vi "CRYAPI TAB LIB.vi"(8 "tPage":T1, 9 "tFrame":T3, 10 "nData":i32, 11 "sAction":string) -> (0 "nData_Out":i32, 2 "tFrame_Out":T3, 3 "tPage_Out":T1)   [LabVIEW 2013]
uses:
  <vilib>/Utility/miscctls.llb/LVRectTypeDef.ctl
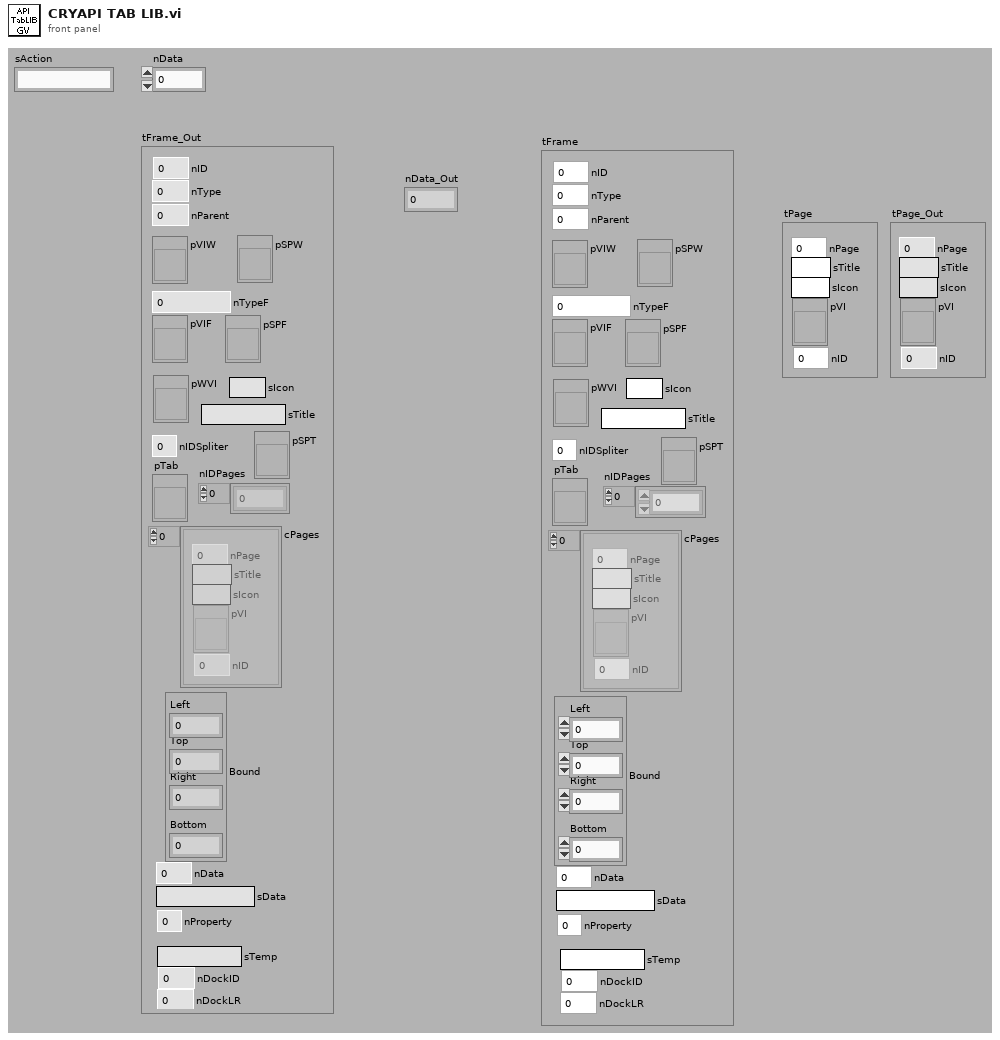
[diagram p1: front panel]
types:
  T1 = cluster{"nPage":i32, "sTitle":string, "sIcon":string, "pVI":refnum<vi>, "nID":i32}
  T2 = typedef "LVRectTypeDef.ctl" = cluster{"Left":i16, "Top":i16, "Right":i16, "Bottom":i16}
  T3 = cluster{"nType":i32, "nParent":i32, "pVIW":refnum<vi>, "pSPW":refnum<vi>, "nTypeF":i32, "pVIF":refnum<vi>, "pSPF":refnum<vi>, "nIDSpliter":i32, "nProperty":i32, "Bound":T2, "nID":i32, "nData":i32, "sData":string, "pWVI":refnum<vi>, "sTitle":string, "cPages":cluster{"nPage":i32, "sTitle":string, "sIcon":string, "pVI":refnum<vi>, "nID":i32}[], "pTab":refnum<vi>, "nIDPages":i32[], "pSPT":refnum<vi>, "sTemp":string, "nDockID":i32, "nDockLR":i32, "sIcon":string}
  T4 = cluster{"nPage":i32, "sTitle":string, "sIcon":string, "pVI":refnum<vi>, "nID":i32}[]
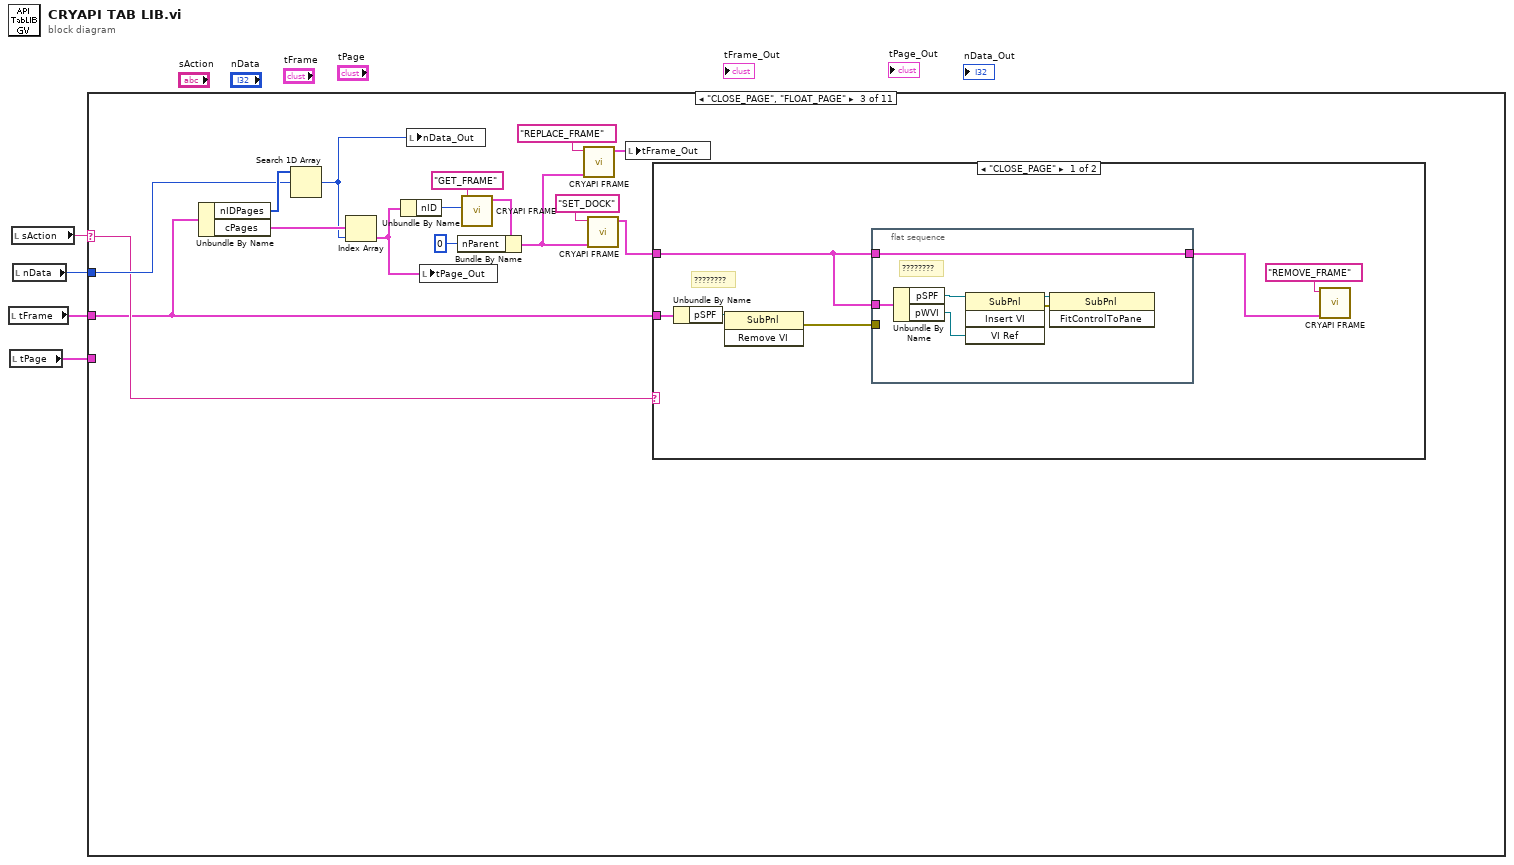
[diagram p0: block diagram]
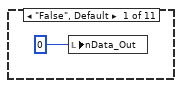
[diagram p2: hidden frame]
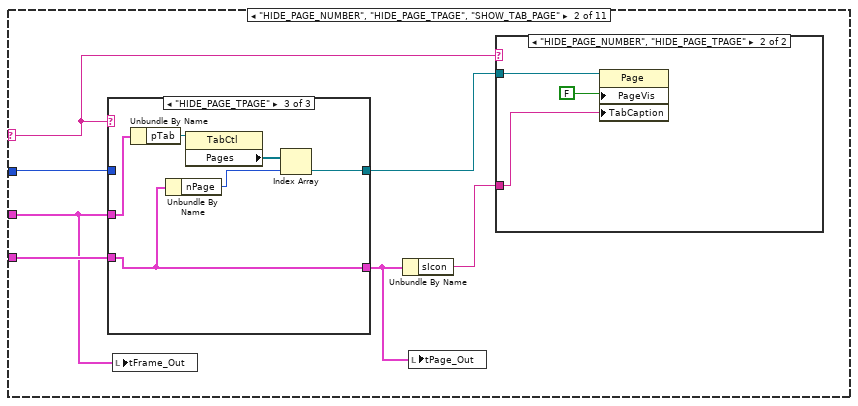
[diagram p3: hidden frame]
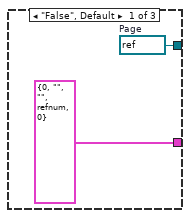
[diagram p4: hidden frame]
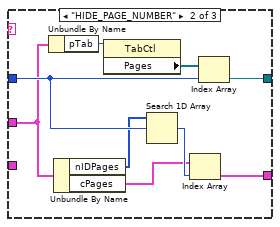
[diagram p5: hidden frame]
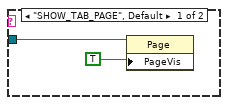
[diagram p6: hidden frame]
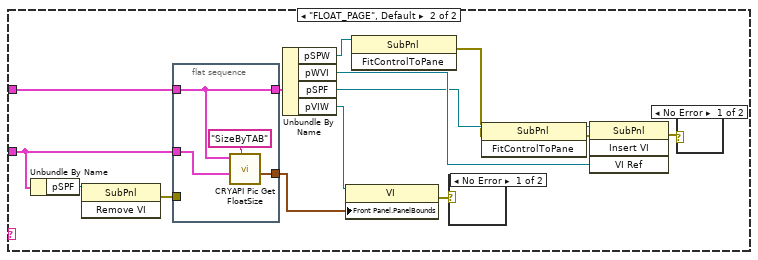
[diagram p7: hidden frame]
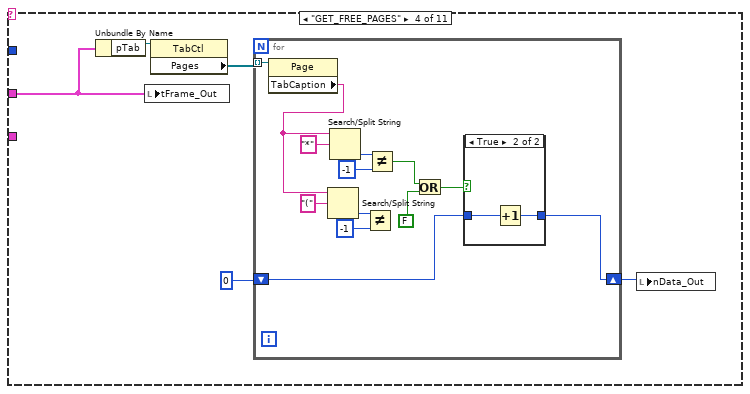
[diagram p10: hidden frame]
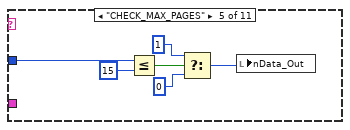
[diagram p12: hidden frame]
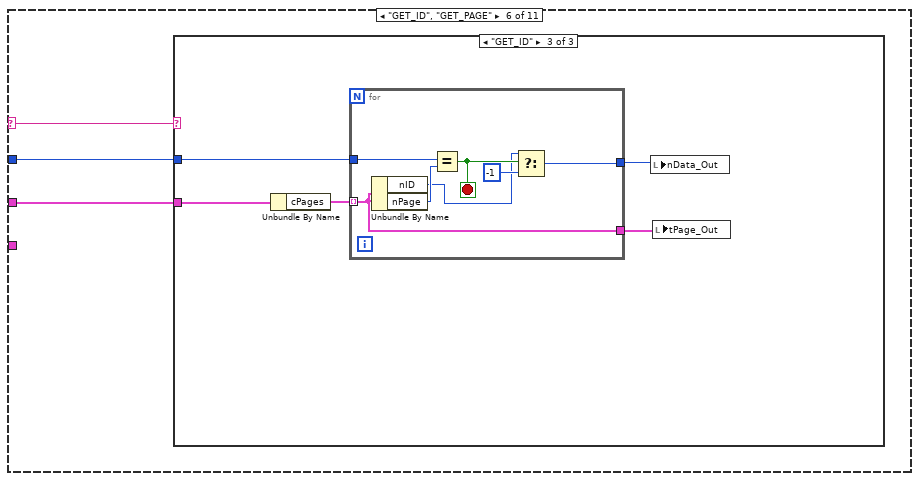
[diagram p13: hidden frame]
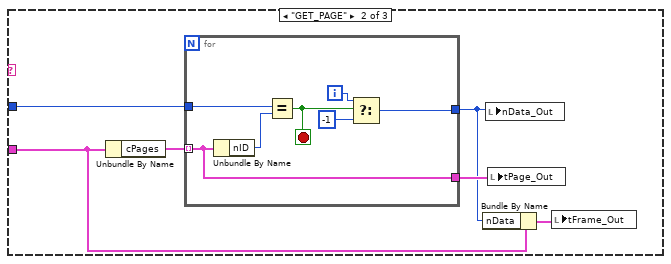
[diagram p15: hidden frame]
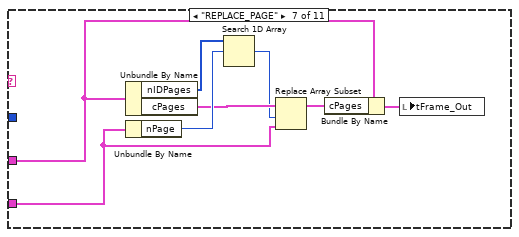
[diagram p16: hidden frame]
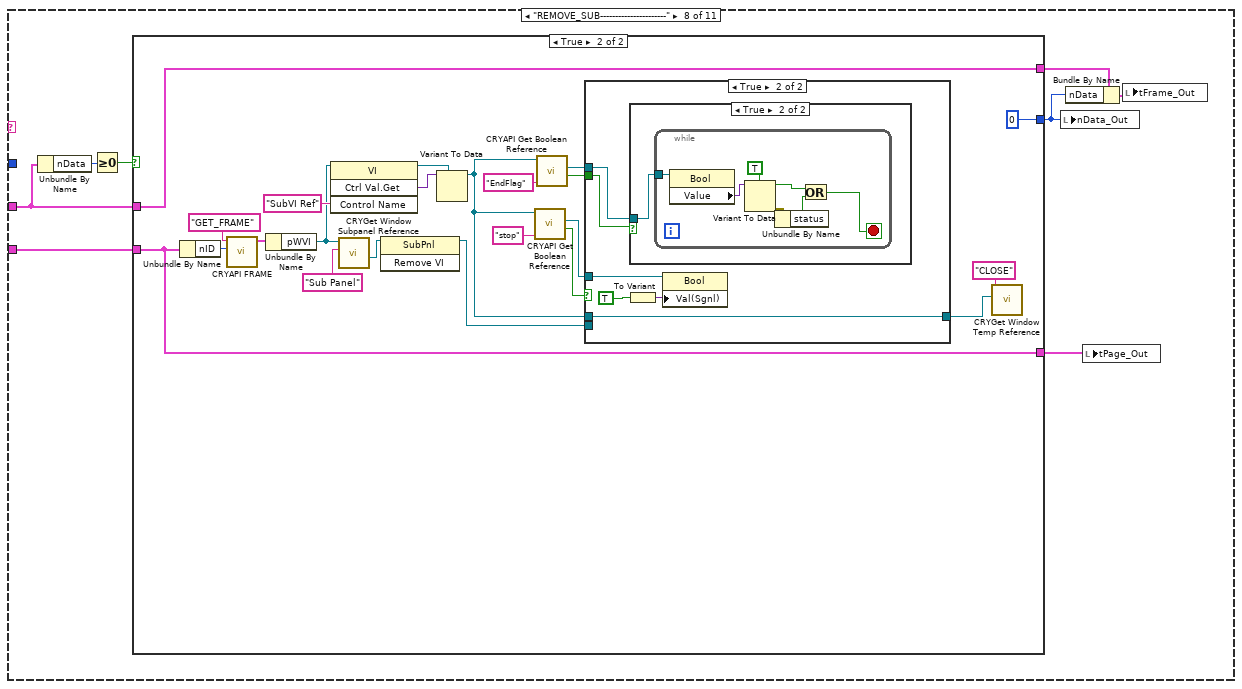
[diagram p17: hidden frame]
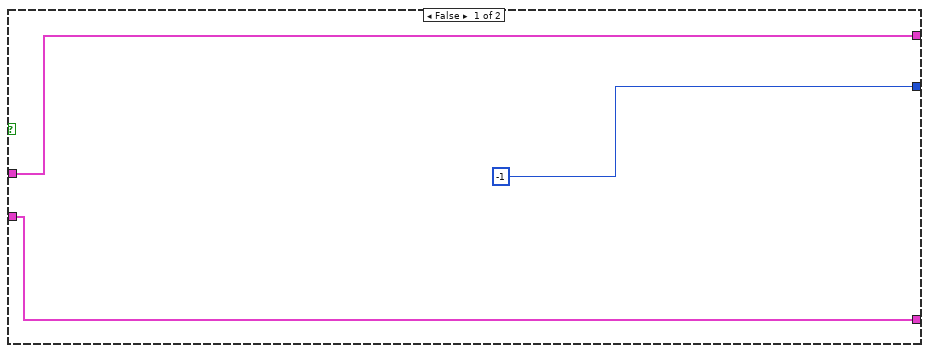
[diagram p18: hidden frame]
diagram:
  n1 = local read "tFrame"() -> (w3:T3)
  n2 = local read "tPage"() -> (w2:T1)
  n3 = local read "sAction"() -> (w4:string)
  n4 = local read "nData"() -> (w1:i32)
  n5 = case shown="\"CLOSE_PAGE\", \"FLOAT_PAGE\"" w4 {
    selector: w4 -> [_ w8 w40 _ _ w109 _ _ _ _ _]
    tunnel: w3 -> [_ w6 w35 w82 _ w110 w142 w146 w194 w258 w288]
    tunnel: w2 -> [_ w7 _ _ _ _ w139 w151 w197 _ _]
    tunnel: w1 -> [_ w11 w47 _ w108 w111 _ _ _ w257 _]
    frame "False", Default {
      n6 = local write "nData_Out"(0 ("nData_Out")) -> ()
    }
    frame "HIDE_PAGE_NUMBER", "HIDE_PAGE_TPAGE", "SHOW_TAB_PAGE" {
      n7 = case shown="\"HIDE_PAGE_TPAGE\"" w8 {
        tunnel: [w14 w21 w27] -> w12
        tunnel: w11 -> [_ w20 _]
        tunnel: [T1 {"nPage"=0, "sTitle"="", "sIcon"="", "pVI"=refnum, "nID"=0} ("tPage") w19 w26] -> w9
        tunnel: w7 -> [_ _ w26]
        tunnel: w6 -> [_ w15 w24]
        frame "False", Default {
          w14 = refnum<vi> refnum  # Page
        }
        frame "HIDE_PAGE_NUMBER" {
          n8 = Unbundle By Name(w15) -> ("pTab"=w23:refnum<vi>)
          n9 = Unbundle By Name(w15) -> ("nIDPages"=w18:i32[], "cPages"=w16:T4)
          n10 = property class="TabCtl"(reference=w23) -> ("Pages"=w22:refnum<vi>[])  [unwired: 1 in, 2 out]
          n11 = Search 1D Array(1D array=w18, element=w20) -> (index of element=w17:i32)  [unwired: 1 out]
          n12 = Index Array(array=w16, index=w17) -> (element=w19:T1)
          n13 = Index Array(array=w22, index=w20) -> (element=w21:refnum<vi>)
        }
        frame "HIDE_PAGE_TPAGE" {
          n14 = Unbundle By Name(w24) -> ("pTab"=w29:refnum<vi>)
          n15 = Unbundle By Name(w26) -> ("nPage"=w25:i32)
          n16 = property class="TabCtl"(reference=w29) -> ("Pages"=w28:refnum<vi>[])  [unwired: 1 in, 2 out]
          n17 = Index Array(array=w28, index=w25) -> (element=w27:refnum<vi>)
        }
      }
      n18 = local write "tFrame_Out"(w6) -> ()
      n19 = Unbundle By Name(w9) -> ("sIcon"=w10:string)
      n20 = local write "tPage_Out"(w9) -> ()
      n21 = case shown="\"HIDE_PAGE_NUMBER\", \"HIDE_PAGE_TPAGE\"" w8 {
        tunnel: w12 -> [w30 w33]
        tunnel: w10 -> [_ w32]
        frame "SHOW_TAB_PAGE", Default {
          n22 = property class="Page"(reference=w30, "PageVis"=TRUE ("Page Visible")) -> ()  [unwired: 1 in, 2 out]
        }
        frame "HIDE_PAGE_NUMBER", "HIDE_PAGE_TPAGE" {
          n23 = property class="Page"(reference=w33, "PageVis"=FALSE ("Page Visible"), "TabCaption"=w32) -> ()  [unwired: 1 in, 2 out]
        }
      }
    }
    frame "CLOSE_PAGE", "FLOAT_PAGE" {
      n24 = Unbundle By Name(w35) -> ("nIDPages"=w49:i32[], "cPages"=w48:T4)
      n25 = Search 1D Array(1D array=w49, element=w47) -> (index of element=w37:i32)  [unwired: 1 out]
      n26 = Index Array(array=w48, index=w37) -> (element=w45:T1)
      n27 = Unbundle By Name(w45) -> ("nID"=w46:i32)
      n28 = local write "nData_Out"(w37) -> ()
      n29 = local write "tPage_Out"(w45) -> ()
      n30 = call "CRYAPI FRAME.vi"("nData"=w46, "sAction"="GET_FRAME") -> ("tFrame_Out"=w44:T3)  [unwired: 4 in, 5 out]
      n31 = Bundle By Name(cluster=w44, "nParent"=0) -> (w38:T3)
      n32 = call "CRYAPI FRAME.vi"("tFrame"=w38, "sAction"="REPLACE_FRAME") -> ("tFrame_Out"=w41:T3)  [unwired: 4 in, 5 out]
      n33 = call "CRYAPI FRAME.vi"("tFrame"=w38, "sAction"="SET_DOCK") -> ("tFrame_Out"=w36:T3)  [unwired: 4 in, 5 out]
      n34 = local write "tFrame_Out"(w41) -> ()
      n35 = case shown="\"CLOSE_PAGE\"" w40 {
        tunnel: w36 -> [w55 w75]
        tunnel: w35 -> [w52 w76]
        frame "CLOSE_PAGE" {
          # "????????"
          n36 = Unbundle By Name(w52) -> ("pSPF"=w53:refnum<vi>)
          n37 = invoke class="SubPnl" method="Remove VI"(reference=w53) -> (error out=w51:errorcluster)  [unwired: 2 in, 2 out]
          n38 = flat-sequence {
            tunnel: w55 -> [w62]
            tunnel: w55 -> [w57]
            tunnel: [w57] -> w54
            tunnel: w51 -> [_]
            frame #0 {
              # "????????"
              n39 = Unbundle By Name(w62) -> ("pSPF"=w59:refnum<vi>, "pWVI"=w58:refnum<vi>)
              n40 = invoke class="SubPnl" method="Insert VI"(reference=w59, "VI Ref"=w58) -> (reference out=w61:refnum<vi>, error out=w60:errorcluster)  [unwired: 2 in, 2 out]
              n41 = invoke class="SubPnl" method="FitControlToPane"(reference=w61, error in=w60) -> ()  [unwired: 1 in, 3 out]
            }
          }
          n42 = call "CRYAPI FRAME.vi"("tFrame"=w54, "sAction"="REMOVE_FRAME") -> ()  [unwired: 4 in, 6 out]
        }
        frame "FLOAT_PAGE", Default {
          n43 = Unbundle By Name(w76) -> ("pSPF"=w77:refnum<vi>)
          n44 = invoke class="SubPnl" method="Remove VI"(reference=w77) -> (error out=w73:errorcluster)  [unwired: 2 in, 2 out]
          n45 = flat-sequence {
            tunnel: w76 -> [w81]
            tunnel: w75 -> [w78]
            tunnel: [w80] -> w74
            tunnel: w73 -> [_]
            tunnel: [w78] -> w72
            frame #0 {
              n46 = call "CRYAPI Pic Get FloatSize.vi"("sAction"="SizeByTAB", "tFrameTAB"=w81, "tFrame"=w78) -> ("FPPanelBound_Out"=w80:T2)  [unwired: 7 in, 1 out]
            }
          }
          n47 = Unbundle By Name(w72) -> ("pSPW"=w65:refnum<vi>, "pWVI"=w70:refnum<vi>, "pSPF"=w68:refnum<vi>, "pVIW"=w71:refnum<vi>)
          n48 = property class="VI"(reference=w71, "Front Panel.PanelBounds"=w74) -> (error out=w63:errorcluster)  [unwired: 1 in, 1 out]
          n49 = invoke class="SubPnl" method="FitControlToPane"(reference=w65) -> (error out=w64:errorcluster)  [unwired: 2 in, 2 out]
          n50 = case shown="No Error" w63 {
            frame No Error {
            }
            frame Error {
            }
          }
          n51 = invoke class="SubPnl" method="FitControlToPane"(reference=w68, error in=w64) -> (reference out=w67:refnum<vi>, error out=w66:errorcluster)  [unwired: 1 in, 1 out]
          n52 = invoke class="SubPnl" method="Insert VI"(reference=w67, error in=w66, "VI Ref"=w70) -> (error out=w69:errorcluster)  [unwired: 1 in, 3 out]
          n53 = case shown="No Error" w69 {
            frame No Error {
            }
            frame Error {
            }
          }
        }
      }
    }
    frame "GET_FREE_PAGES" {
      n54 = Unbundle By Name(w82) -> ("pTab"=w86:refnum<vi>)
      n55 = local write "tFrame_Out"(w82) -> ()
      n56 = property class="TabCtl"(reference=w86) -> ("Pages"=w85:refnum<vi>[])  [unwired: 1 in, 2 out]
      n57 = for {
        tunnel: w85 -> [w99] mode=indexing
        shift-right: [w88] -> w83
        shift-left: 0 -> [w89]
        n58 = property class="Page"(reference=w99) -> ("TabCaption"=w92:string)  [unwired: 1 in, 2 out]
        n59 = Search/Split String(string=w92, search string/char (-)="(") -> (offset of match=w95:i32)  [unwired: 3 out]
        n60 = Search/Split String(string=w92, search string/char (-)="*") -> (offset of match=w97:i32)  [unwired: 3 out]
        n61 = Not Equal?(x=w95, y=-1) -> ()  [unwired: 1 out]
        n62 = Not Equal?(x=w97, y=-1) -> (x != y?=w91:bool)
        n63 = Or(x=w91, y=FALSE) -> (x .or. y?=w90:bool)
        n64 = case shown="True" w90 {
          tunnel: w89 -> [w100 w102]
          tunnel: [w100 w101] -> w88
          frame False {
          }
          frame True {
            n65 = Increment(x=w102) -> (x+1=w101:i32)
          }
        }
      }
      n66 = local write "nData_Out"(w83) -> ()
    }
    frame "CHECK_MAX_PAGES" {
      n67 = Less Or Equal?(x=w108, y=15) -> (x <= y?=w106:bool)
      n68 = Select(t=1, s=w106, f=0) -> (s? t:f=w103:i32)
      n69 = local write "nData_Out"(w103) -> ()
    }
    frame "GET_ID", "GET_PAGE" {
      n70 = case shown="\"GET_ID\"" w109 {
        tunnel: w111 -> [_ w116 w128]
        tunnel: w110 -> [_ w114 w126]
        frame "False", Default {
        }
        frame "GET_PAGE" {
          n71 = Unbundle By Name(w114) -> ("cPages"=w117:T4)
          n72 = for {
            tunnel: w117 -> [w122] mode=indexing
            tunnel: w116 -> [w124]
            tunnel: [w122] -> w115
            tunnel: [w118] -> w113
            i -> [w120]
            stop <- w121 stop-if-true
            n73 = Unbundle By Name(w122) -> ("nID"=w123:i32)
            n74 = Equal?(x=w124, y=w123) -> (x = y?=w121:bool)
            n75 = Select(t=w120, s=w121, f=-1) -> (s? t:f=w118:i32)
          }
          n76 = Bundle By Name(cluster=w114, "nData"=w113) -> (w112:T3)
          n77 = local write "nData_Out"(w113) -> ()
          n78 = local write "tPage_Out"(w115) -> ()
          n79 = local write "tFrame_Out"(w112) -> ()
        }
        frame "GET_ID" {
          n80 = Unbundle By Name(w126) -> ("cPages"=w129:T4)
          n81 = for {
            tunnel: w129 -> [w134] mode=indexing
            tunnel: w128 -> [w136]
            tunnel: [w134] -> w127
            tunnel: [w131] -> w125
            stop <- w133 stop-if-true
            n82 = Unbundle By Name(w134) -> ("nID"=w130:i32, "nPage"=w135:i32)
            n83 = Equal?(x=w136, y=w135) -> (x = y?=w133:bool)
            n84 = Select(t=w130, s=w133, f=-1) -> (s? t:f=w131:i32)
          }
          n85 = local write "nData_Out"(w125) -> ()
          n86 = local write "tPage_Out"(w127) -> ()
        }
      }
    }
    frame "REPLACE_PAGE" {
      n87 = Unbundle By Name(w142) -> ("nIDPages"=w144:i32[], "cPages"=w141:T4)
      n88 = Unbundle By Name(w139) -> ("nPage"=w143:i32)
      n89 = Search 1D Array(1D array=w144, element=w143) -> (index of element=w140:i32)  [unwired: 1 out]
      n90 = Replace Array Subset(array=w141, new element=w139, index=w140) -> (w138:T4)
      n91 = Bundle By Name(cluster=w142, "cPages"=w138) -> (w137:T3)
      n92 = local write "tFrame_Out"(w137) -> ()
    }
    frame "REMOVE_SUB----------------------" {
      n93 = Unbundle By Name(w146) -> ("nData"=w145:i32)
      n94 = Greater Or Equal To 0?(x=w145) -> (x >= 0?=w152:bool)
      n95 = case shown="True" w152 {
        tunnel: w146 -> [w154 w176]
        tunnel: w151 -> [w153 w175]
        tunnel: [-1 ("nData_Out") 0 ("nData_Out")] -> w148
        tunnel: [w154 w176] -> w149
        tunnel: [w153 w175] -> w150
        frame False {
        }
        frame True {
          n96 = Unbundle By Name(w175) -> ("nID"=w173:i32)
          n97 = call "CRYAPI FRAME.vi"("nData"=w173, "sAction"="GET_FRAME") -> ("tFrame_Out"=w165:T3)  [unwired: 4 in, 5 out]
          n98 = Unbundle By Name(w165) -> ("pWVI"=w169:refnum<vi>)
          n99 = invoke class="VI" method="Ctrl Val.Get"(reference=w169, "Control Name"="SubVI Ref" ("Label Name")) -> ("Get Control Value Variant"=w170:variant)  [unwired: 2 in, 3 out]
          n100 = call "CRYGet Window Subpanel Reference.vi"("Sub Panel Name"="Sub Panel", "VI Ref In"=w169) -> ("SubPnl Refnum"=w167:refnum<vi>)  [unwired: 9 out]
          n101 = invoke class="SubPnl" method="Remove VI"(reference=w167) -> (reference out=w160:refnum<vi>)  [unwired: 2 in, 2 out]
          n102 = Variant To Data(type=w169, Variant=w170) -> (data=w161:refnum<vi>)  [unwired: 1 in, 1 out]
          n103 = call "CRYAPI Get Boolean Reference.vi"("Label Name"="stop", "VI Refnum"=w161) -> ("Boolean"=w159:bool, "Boolean Ref"=w158:refnum<vi>)  [unwired: 8 out]
          n104 = call "CRYAPI Get Boolean Reference.vi"("Label Name"="EndFlag", "VI Refnum"=w161) -> ("Boolean"=w157:bool, "Boolean Ref"=w156:refnum<vi>)  [unwired: 8 out]
          n105 = case shown="True" w159 {
            tunnel: w158 -> [_ w182]
            tunnel: w161 -> [w177 w180]
            tunnel: [w177 w180] -> w162
            tunnel: w160 -> [_ _]
            tunnel: w157 -> [_ w179]
            tunnel: w156 -> [_ w178]
            frame False {
            }
            frame True {
              n106 = To Variant(anything=TRUE) -> (Variant=w181:variant)
              n107 = case shown="True" w179 {
                tunnel: w178 -> [_ w184]
                frame False {
                }
                frame True {
                  n108 = while {
                    tunnel: w184 -> [w191]
                    stop <- w185 stop-if-true
                    n109 = property class="Bool"(reference=w191) -> ("Value"=w190:variant)  [unwired: 1 in, 2 out]
                    n110 = Variant To Data(type=TRUE, Variant=w190) -> (data=w186:bool, error out=w188:errorcluster)  [unwired: 1 in]
                    n111 = Unbundle By Name(w188) -> ("status"=w187:bool)
                    n112 = Or(x=w186, y=w187) -> (x .or. y?=w185:bool)
                  }
                }
              }
              n113 = property class="Bool"(reference=w182, "Val(Sgnl)"=w181) -> ()  [unwired: 1 in, 2 out]
            }
          }
          n114 = call "CRYGet Window Temp Reference.vi"("pVIRef_In"=w162, "sAction"="CLOSE") -> ()  [unwired: 2 in, 8 out]
        }
      }
      n115 = local write "nData_Out"(w148) -> ()
      n116 = Bundle By Name(cluster=w149, "nData"=w148) -> (w147:T3)
      n117 = local write "tPage_Out"(w150) -> ()
      n118 = local write "tFrame_Out"(w147) -> ()
    }
    frame "RESET_SUB" {
      n119 = Unbundle By Name(w194) -> ("nData"=w193:i32)
      n120 = Greater Or Equal To 0?(x=w193) -> (x >= 0?=w198:bool)
      n121 = case shown="True" w198 {
        tunnel: w194 -> [w200 w213]
        tunnel: w197 -> [_ w218]
        tunnel: [w200 w213] -> w196
        tunnel: [0 ("nData_Out") w206] -> w192
        frame False {
        }
        frame True {
          n122 = Unbundle By Name(w218) -> ("nID"=w215:i32)
          n123 = call "CRYAPI FRAME.vi"("nData"=w215, "sAction"="GET_FRAME") -> ("tFrame_Out"=w216:T3)  [unwired: 4 in, 5 out]
          n124 = Unbundle By Name(w213) -> ("pWVI"=w214:refnum<vi>)
          n125 = Unbundle By Name(w216) -> ("nID"=w206:i32, "pWVI"=w205:refnum<vi>)
          n126 = stacked-sequence {
            tunnel: w205 -> [w229]
            tunnel: [w229] -> w202
            frame #0 {
              n127 = call "CRYAPI FILE.vi"("sData"="RESET_SUB:TAB", "sAction"="OUT_LOG") -> ()  [unwired: 8 in, 2 out]
            }
          }
          n128 = while {
            tunnel: w214 -> [w224]
            tunnel: w202 -> [w223]
            tunnel: [w219] -> w201
            stop <- w221 stop-if-true
            n129 = To Variant(anything=w224) -> (Variant=w225:variant)
            n130 = invoke class="VI" method="Ctrl Val.Set"(reference=w223, "Control Name"="SubVI Ref" ("Label Name"), "Value"=w225) -> (reference out=w219:refnum<vi>, error out=w222:errorcluster)  [unwired: 2 in, 3 out]
            n131 = case shown="Error" w222 {
              tunnel: [TRUE FALSE] -> w221
              frame No Error {
              }
              frame Error {
              }
            }
            n132 = Wait Until Next ms Multiple(millisecond multiple=u32 10) -> ()  [unwired: 1 out]
          }
          n133 = flat-sequence {
            tunnel: w214 -> [w237]
            tunnel: [w237] -> w204
            tunnel: [w236] -> w203
            tunnel: w201 -> [w235]
            tunnel: [w238] -> w211
            tunnel: [w241] -> w212
            tunnel: w204 -> [w241]
            tunnel: w203 -> [w239]
            tunnel: [w245] -> w210
            tunnel: [w247] -> w209
            tunnel: w212 -> [w243]
            tunnel: w211 -> [w246]
            tunnel: w210 -> [w251]
            tunnel: [w249] -> w208
            tunnel: [w248] -> w207
            tunnel: w209 -> [w250]
            tunnel: w208 -> [w256]
            tunnel: w207 -> [w255]
            frame #0 {
              n134 = call "CRYGet Window Subpanel Reference.vi"("Sub Panel Name"="Sub Panel", "VI Ref In"=w235) -> ("SubPnl Refnum"=w236:refnum<vi>)  [unwired: 9 out]
              n135 = call "CRYAPI FILE.vi"("sData"="RESET_SUB:GET", "sAction"="OUT_LOG") -> ()  [unwired: 8 in, 2 out]
            }
            frame #1 {
              n136 = property class="SubPnl"(reference=w239, "Visible"=FALSE) -> (reference out=w238:refnum<vi>)  [unwired: 1 in, 1 out]
            }
            frame #2 {
              n137 = invoke class="VI" method="Run VI"(reference=w243, "Wait until done"=FALSE ("Wait Until Done")) -> (reference out=w242:refnum<vi>)  [unwired: 3 in, 4 out]
              n138 = invoke class="SubPnl" method="Insert VI"(reference=w246, "VI Ref"=w242) -> (reference out=w245:refnum<vi>, error out=w247:errorcluster)  [unwired: 2 in, 2 out]
            }
            frame #3 {
              n139 = invoke class="SubPnl" method="FitControlToPane"(reference=w251, error in=w250) -> (reference out=w249:refnum<vi>, error out=w248:errorcluster)  [unwired: 1 in, 1 out]
            }
            frame #4 {
              n140 = property class="SubPnl"(reference=w256, error in=w255, "Visible"=TRUE) -> ()  [unwired: 2 out]
              n141 = call "CRYAPI FILE.vi"("sData"="RESET_SUB:OK", "sAction"="OUT_LOG") -> ()  [unwired: 8 in, 2 out]
            }
          }
        }
      }
      n142 = Bundle By Name(cluster=w196, "nData"=w192) -> (w195:T3)
      n143 = local write "nData_Out"(w192) -> ()
      n144 = local write "tFrame_Out"(w195) -> ()
    }
    frame "GET_PAGE_WID" {
      n145 = Unbundle By Name(w258) -> ("cPages"=w259:T4)
      n146 = for {
        tunnel: w259 -> [w269] mode=indexing
        tunnel: w257 -> [w268]
        shift-right: [w262] -> w261
        shift-left: -1 -> [w263]
        stop <- w264 stop-if-true
        n147 = Unbundle By Name(w269) -> ("nID"=w267:i32, "nPage"=w265:i32)
        n148 = Equal?(x=w268, y=w267) -> (x = y?=w266:bool)
        n149 = case shown="True" w266 {
          selector: w266 -> [w271 w273]
          tunnel: w265 -> [_ w272]
          tunnel: [w271 w273] -> w264
          tunnel: w263 -> [w270 _]
          tunnel: [w270 w272] -> w262
          frame False {
          }
          frame True {
          }
        }
      }
      n150 = local write "nData_Out"(w261) -> ()
    }
    frame "PAGE_IS_GRAPH_WINDOW" {
      n151 = Unbundle By Name(w288) -> ("cPages"=w287:T4, "pTab"=w286:refnum<vi>)
      n152 = property class="TabCtl"(reference=w286) -> ("Value"=w285:variant)  [unwired: 1 in, 2 out]
      n153 = Variant To Data(type=0, Variant=w285) -> (data=w283:i32)  [unwired: 1 in, 1 out]
      n154 = for {
        tunnel: w287 -> [w315] mode=indexing
        tunnel: w283 -> [w313]
        shift-right: [w309] -> w281
        shift-left: -1 -> [w311]
        tunnel: [w307] -> w280
        tunnel: [w306] -> w279
        i -> [w310]
        stop <- w308 stop-if-true
        n155 = Unbundle By Name(w315) -> ("nID"=w306:i32, "pVI"=w307:refnum<vi>, "nPage"=w314:i32)
        n156 = Equal?(x=w314, y=w313) -> (x = y?=w312:bool)
        n157 = case shown="False" w312 {
          selector: w312 -> [w316 w318]
          tunnel: w311 -> [w317 _]
          tunnel: w310 -> [_ w319]
          tunnel: [w317 w319] -> w309
          tunnel: [w316 w318] -> w308
          frame False {
          }
          frame True {
          }
        }
      }
      n158 = case shown="Default" w281 {
        tunnel: w280 -> [w291 _]
        tunnel: w279 -> [w294 _]
        tunnel: [w290 FALSE ("Is Display Step?")] -> w277
        tunnel: [w289 _] -> w278
        frame Default {
          n159 = call "CRYAPI FRAME.vi"("nData"=w294, "sAction"="GET_FRAME") -> ("tFrame_Out"=w289:T3)  [unwired: 6 in, 3 out]
          n160 = Unbundle By Name(w289) -> ("sTemp"=w292:string)
          n161 = call "CRYCheck Sub Data View.vi"("VI Refnum"=w291, "Window Name"=w292) -> ("data view?"=w293:bool)  [unwired: 9 out]
          n162 = case shown="True" w293 {
            tunnel: w292 -> [_ w301]
            tunnel: w291 -> [_ w299]
            tunnel: [FALSE w297] -> w290
            frame False {
            }
            frame True {
              n163 = Equal?(x=w301, y="Step Setup") -> (x = y?=w298:bool)
              n164 = case shown="False" w298 {
                tunnel: w299 -> [_ w304]
                tunnel: [TRUE ("Is Display Step?") w303] -> w297
                frame False {
                }
                frame True {
                  n165 = call "CRYIs Display Step.vi"("pVIF_Out"=w304) -> ("Is Display Step?"=w303:bool)  [unwired: 10 in]
                }
              }
            }
          }
        }
        frame -1 {
        }
      }
      n166 = local write "tFrame_Out"(w278) -> ()
      n167 = Select(t=1, s=w277, f=-1) -> (s? t:f=w274:i32)
      n168 = local write "nData_Out"(w274) -> ()
    }
  }
